vi "数组.vi"() -> ()   [LabVIEW 2014]
panel:
  out "显示整行 2":dbl[](array[numeric])
  out "行 4":i8
  in  "布尔":bool
  out "列 2":i8
  out "行 3":i8
  out "数组 7":i8[][](array[numeric])
  in  "替换值":i8
  in  "列":i8
  in  "行":i8
  in  "菜单下拉列表":u16(ring) items=["替换值1", "替换行"]
  in  "替换行值 2":i8[](array[numeric])
  in  "替换行":i8
  out "数组 6":i8[][](array[numeric])
  in  "行 2":i8
  out "显示整行":i8[](array[numeric])
  out "数值":i8
  in  "列":i8
  in  "行":i8
  out "数组 5":i8[][](array[numeric])
  out "数组结果":i8[](array[numeric])
  out "数组 4":i8[](array[numeric])
  in  "数组 3":i8[][](array[numeric])
  in  "数组 2":bool[](array[boolean])
  in  "数组":i8[](array[numeric])
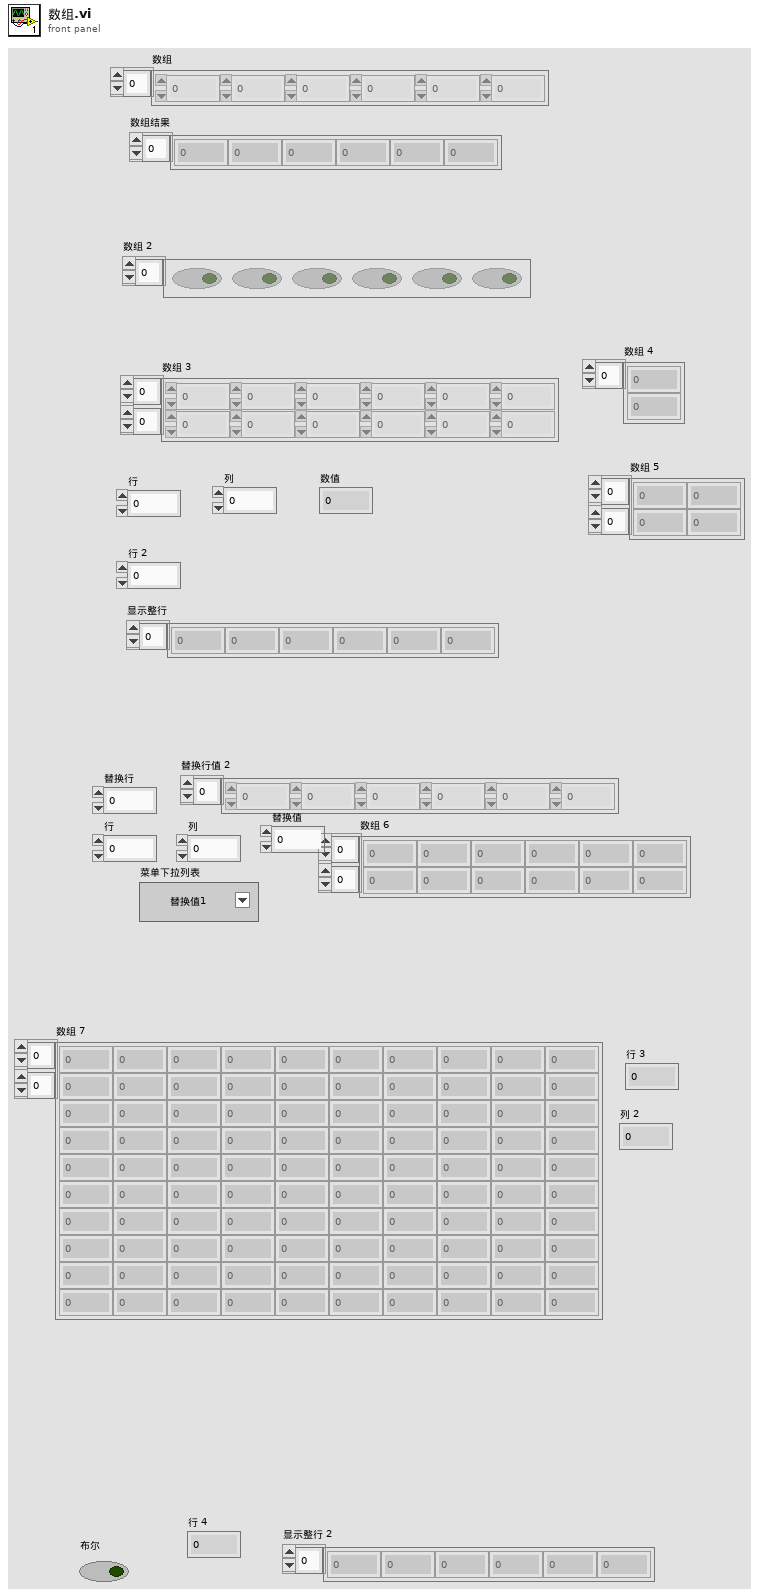
[diagram p1: front panel]
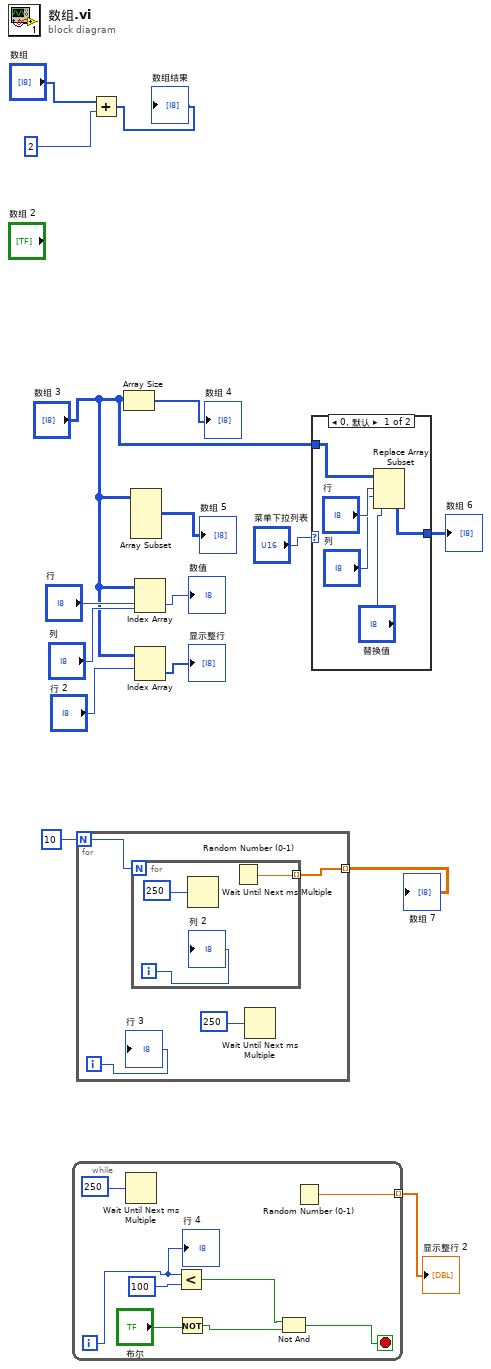
[diagram p0: block diagram]
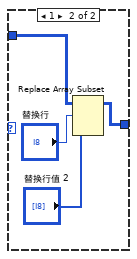
[diagram p2: hidden frame]
diagram:
  n1 = while {
    tunnel: [w17] -> w1 mode=indexing
    i -> [w19]
    stop <- w22 stop-if-true
    n2 = Wait Until Next ms Multiple(millisecond multiple=250) -> ()  [unwired: 1 out]
    n3 = Less?(x=w19, y=100) -> (x < y?=w21:bool)
    n4 = Not(x="布尔") -> (.not. x?=w23:bool)
    n5 = Not And(1:w23, 2:w21) -> (0:w22:bool)
    n6 = Random Number (0-1)() -> (number: 0 to 1=w17:dbl)
    "行 4" <- w19
  }
  "显示整行 2" <- w1
  n7 = for {
    N: 10 -> [w25]
    tunnel: [w27] -> w2 mode=indexing
    i -> [w26]
    n8 = for {
      N: w25 -> [_]
      tunnel: [w30] -> w27 mode=indexing
      i -> [w31]
      n9 = Wait Until Next ms Multiple(millisecond multiple=250) -> ()  [unwired: 1 out]
      n10 = Random Number (0-1)() -> (number: 0 to 1=w30:dbl)
      "列 2" <- w31
    }
    n11 = Wait Until Next ms Multiple(millisecond multiple=250) -> ()  [unwired: 1 out]
    "行 3" <- w26
  }
  "数组 7" <- w2
  n12 = Add(x="数组", y=2) -> (x+y=→"数组结果":i32[])
  n13 = Array Size(array="数组 3") -> (size(s)=→"数组 4":i32[])
  n14 = Array Subset(array="数组 3") -> (→"数组 5":i8[][])  [unwired: 4 in]
  n15 = Index Array(array="数组 3", index (row)="行", index (col)="列") -> (element=→"数值":i8)
  n16 = Index Array(array="数组 3", index (row)="行 2") -> (element=→"显示整行":i8[])  [unwired: 1 in]
  n17 = case shown="0, 默认" "菜单下拉列表" {
    tunnel: [w35 w40] -> w6
    tunnel: "数组 3" -> [w34 w39]
    frame 0, Default {
      n18 = Replace Array Subset(array=w34, new element="替换值", index (row)="行", index (col)="列") -> (w35:i8[][])
    }
    frame 1 {
      n19 = Replace Array Subset(array=w39, new element="替换行值 2", index (row)="替换行") -> (w40:i8[][])  [unwired: 1 in]
    }
  }
  "数组 6" <- w6
